vi "SetSourcePower.vi"(0 "VISA IN":refnum<visa-resource-name>="PNA", 5 "error in":errorcluster) -> (14 "VISA Out":refnum<visa-resource-name>, 19 "error out":errorcluster)   [LabVIEW 2018, in "PNA-X.lvlib"]
uses:
  PNA-X.lvlib
panel:
  in  "PowerLevel":dbl
  in  "Source":string
  in  "Coupling ON/OFF":bool
  in  "Stop Power":dbl
  in  "Start Power":dbl
  in  "Source State":string(combo)
  in  "Atten(db)":dbl=10.0
  in  "Port":i32=1
  in  "AutoRange?":bool
  in  "Channel":i32=1
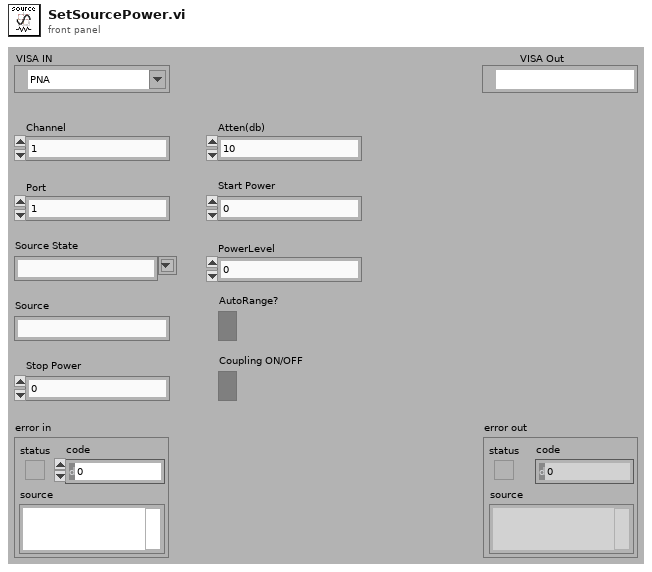
[diagram p1: front panel]
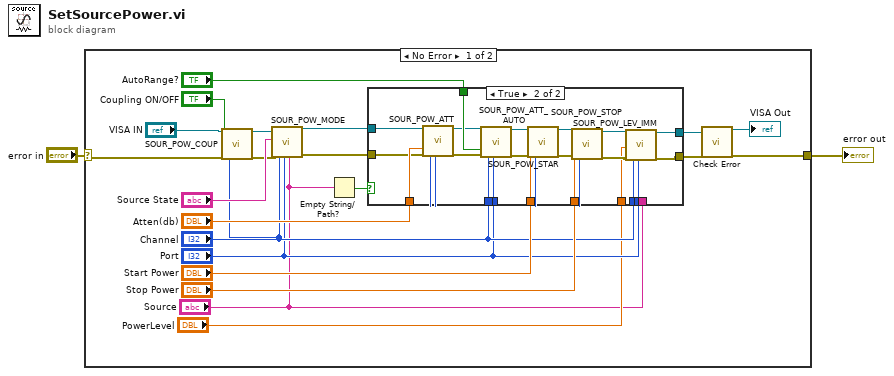
[diagram p0: block diagram]
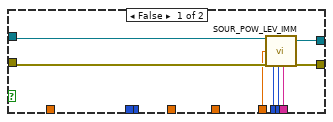
[diagram p2: hidden frame]
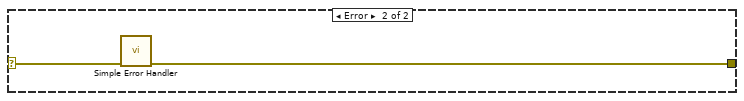
[diagram p3: hidden frame]
diagram:
  n1 = case shown="No Error" "error in" {
    selector: "error in" -> [w17 w54]
    tunnel: [w10 w53] -> w2
    frame No Error {
      n2 = call "SOUR_POW_COUP.vi"("VISA IN"="VISA IN", "Coupling ON/OFF"="Coupling ON/OFF", "error in"=w17, "Channel"="Channel") -> ("VISA Out"=w16:refnum<visa-resource-name>, "error out"=w18:errorcluster)  [unwired: 14 in]
      n3 = call "SOUR_POW_MODE.vi"("VISA IN"=w16, "Source State"="Source State", "error in"=w18, "Channel"="Channel", "Port number"="Port", "Source"="Source") -> ("VISA Out"=w14:refnum<visa-resource-name>, "error out"=w13:errorcluster)  [unwired: 12 in]
      n4 = Empty String/Path?(string/path="Source") -> (empty?=w11:bool)
      n5 = case shown="True" w11 {
        tunnel: "Atten(db)" -> [_ w52]
        tunnel: "AutoRange?" -> [_ w51]
        tunnel: "Port" -> [_ w50]
        tunnel: "Start Power" -> [_ w47]
        tunnel: "Stop Power" -> [_ w46]
        tunnel: "Channel" -> [_ w45]
        tunnel: w14 -> [w28 w44]
        tunnel: w13 -> [w31 w39]
        tunnel: [w30 w37] -> w8
        tunnel: [w29 w35] -> w7
        tunnel: "Channel" -> [w27 w34]
        tunnel: "Port" -> [w26 w33]
        tunnel: "PowerLevel" -> [w25 w32]
        tunnel: "Source" -> [w24 _]
        frame False {
          n6 = call "SOUR_POW_LEV_IMM.vi"("VISA IN"=w28, "Power Level"=w25, "error in"=w31, "Channel"=w27, "Port number"=w26, "Source"=w24) -> ("VISA Out"=w29:refnum<visa-resource-name>, "error out"=w30:errorcluster)  [unwired: 12 in]
        }
        frame True {
          n7 = call "SOUR_POW_ATT.vi"("VISA IN"=w44, "Atten(db)"=w52, "error in"=w39, "Channel"=w45, "Port"=w50) -> ("VISA Out"=w42:refnum<visa-resource-name>, "error out"=w43:errorcluster)  [unwired: 13 in]
          n8 = call "SOUR_POW_ATT_AUTO.vi"("VISA IN"=w42, "Auto?"=w51, "error in"=w43, "Channel"=w45, "Port"=w50) -> ("VISA Out"=w41:refnum<visa-resource-name>, "error out"=w40:errorcluster)  [unwired: 13 in]
          n9 = call "SOUR_POW_STAR.vi"("VISA IN"=w41, "Start Power"=w47, "error in"=w40, "Channel"=w45) -> ("VISA Out"=w48:refnum<visa-resource-name>, "error out"=w49:errorcluster)  [unwired: 14 in]
          n10 = call "SOUR_POW_STOP.vi"("VISA IN"=w48, "Stop Power"=w46, "error in"=w49, "Channel"=w45) -> ("VISA Out"=w36:refnum<visa-resource-name>, "error out"=w38:errorcluster)  [unwired: 14 in]
          n11 = call "SOUR_POW_LEV_IMM.vi"("VISA IN"=w36, "Power Level"=w32, "error in"=w38, "Channel"=w34, "Port number"=w33) -> ("VISA Out"=w35:refnum<visa-resource-name>, "error out"=w37:errorcluster)  [unwired: 13 in]
        }
      }
      n12 = call "Check Error.vi"("VISA Resource Name"=w7, "error in (no error)"=w8) -> ("dup VISA session"=→"VISA Out":refnum<visa-resource-name>, "error out"=w10:errorcluster)  [unwired: 16 in]
    }
    frame Error {
      n13 = call <vilib>:"Simple Error Handler.vi"("error in (no error)"=w54) -> ("error out"=w53:errorcluster)  [unwired: 4 in, 4 out]
    }
  }
  "error out" <- w2
